vi "BASE_Parameters.vi"(8 "error in (no error)":errorcluster) -> (0 "error out":errorcluster)   [LabVIEW 2017]
doc: "this is Hardware setting to set ip address and com port of scanner"
uses:
  Global/PLC_to_Auto.vi
panel:
  in  "System Tab":T1(tab)
  in  "WRITE IN PLC":bool
  in  "MOTOR PARAMETERS":T2={"SPEED 1"=1000, "SPEED 2"=500, "SPEED 3"=100, "DISTANCE 1"=60.0, "DISTANCE 2"=5.0, "DISTANCE 3"=2.0, "MICRO STEP"=8, "STROKE COUNTER"=60} {"STROKE COUNTER" min=15 max=60 step=1; "MICRO STEP" min=1 max=3 step=1; "DISTANCE 3" min=0.5 max=2 step=0.1 format="%#.1g"; "DISTANCE 2" min=1 max=5 step=0.1 format="%#.1g"; "DISTANCE 1" min=40 max=60 step=0.1 format="%#.1g"; "SPEED 3" min=50 max=100 step=1; "SPEED 2" min=300 max=500 step=1; "SPEED 1" min=1000 max=2000 step=1}
  in  "TF CHECKING PARAMATERS":T3={"TRIP FORCE MIN"=40, "RESET FORCE MIN"=350, "OFFSET"=10, "TRIP FORCE MAX"=40, "RESET FORCE MAX"=350} {"RESET FORCE MAX" min=200 max=350 step=1; "TRIP FORCE MAX" min=15 max=40 step=1; "OFFSET" min=-10 max=10 step=1; "RESET FORCE MIN" min=200 max=350 step=1; "TRIP FORCE MIN" min=15 max=40 step=1}
  in  "Save Button":bool
  in  "Back":bool
  # "BARCODE VERIFICATION SYSTEM REPORTS"
  # "SPEED 1\t2000\nSPEED 2\t300\nSPEED 3\t100\nDISTANCE 1\t77.5 MM\nDISTANCE 2\t1.5 MM\nDISTANCE 3\t1.2 MM\nMEASURE BY MICRO\t5"
  # "Parameter Setting"
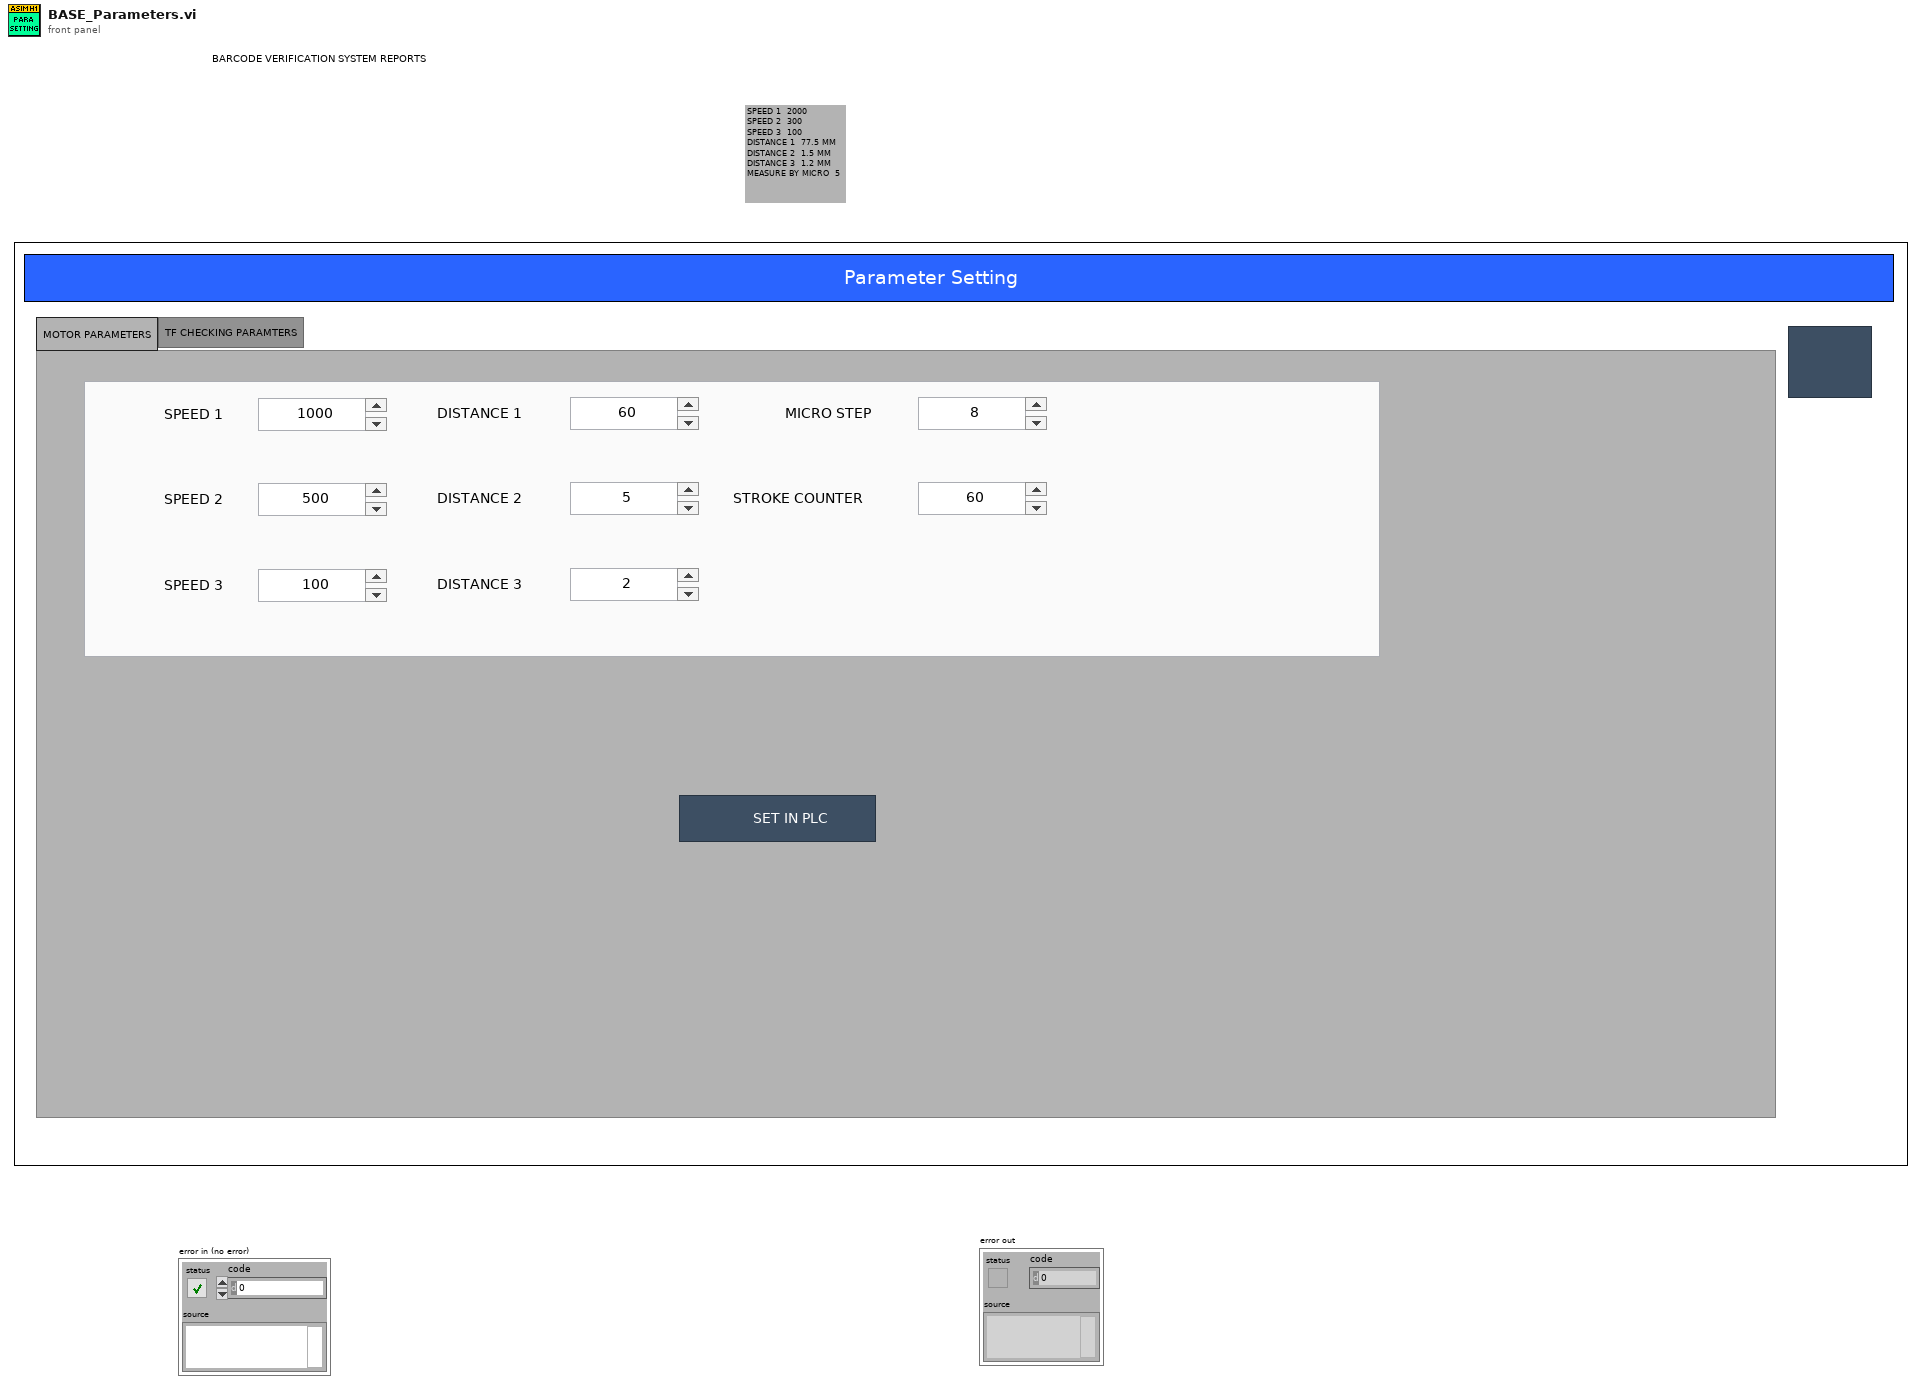
[diagram p1: front panel]
types:
  T1 = enum32{"MOTOR PARAMETERS", "TF CHECKING PARAMTERS"}
  T2 = cluster{"SPEED 1":u16, "SPEED 2":u16, "SPEED 3":u16, "DISTANCE 1":sgl, "DISTANCE 2":sgl, "DISTANCE 3":sgl, "MICRO STEP":u16, "STROKE COUNTER":u16}
  T3 = cluster{"TRIP FORCE MIN":u16, "RESET FORCE MIN":u16, "OFFSET":i16, "TRIP FORCE MAX":u16, "RESET FORCE MAX":u16}
  T4 = enum32{"invalid app kind", "Development System", "Run Time System", "Student Edition", "Embedded LabVIEW", "Evaluation", "Custom"}
  T5 = enum32{"Invalid", "Standard", "Closed", "Hidden", "Minimized", "Maximized"}
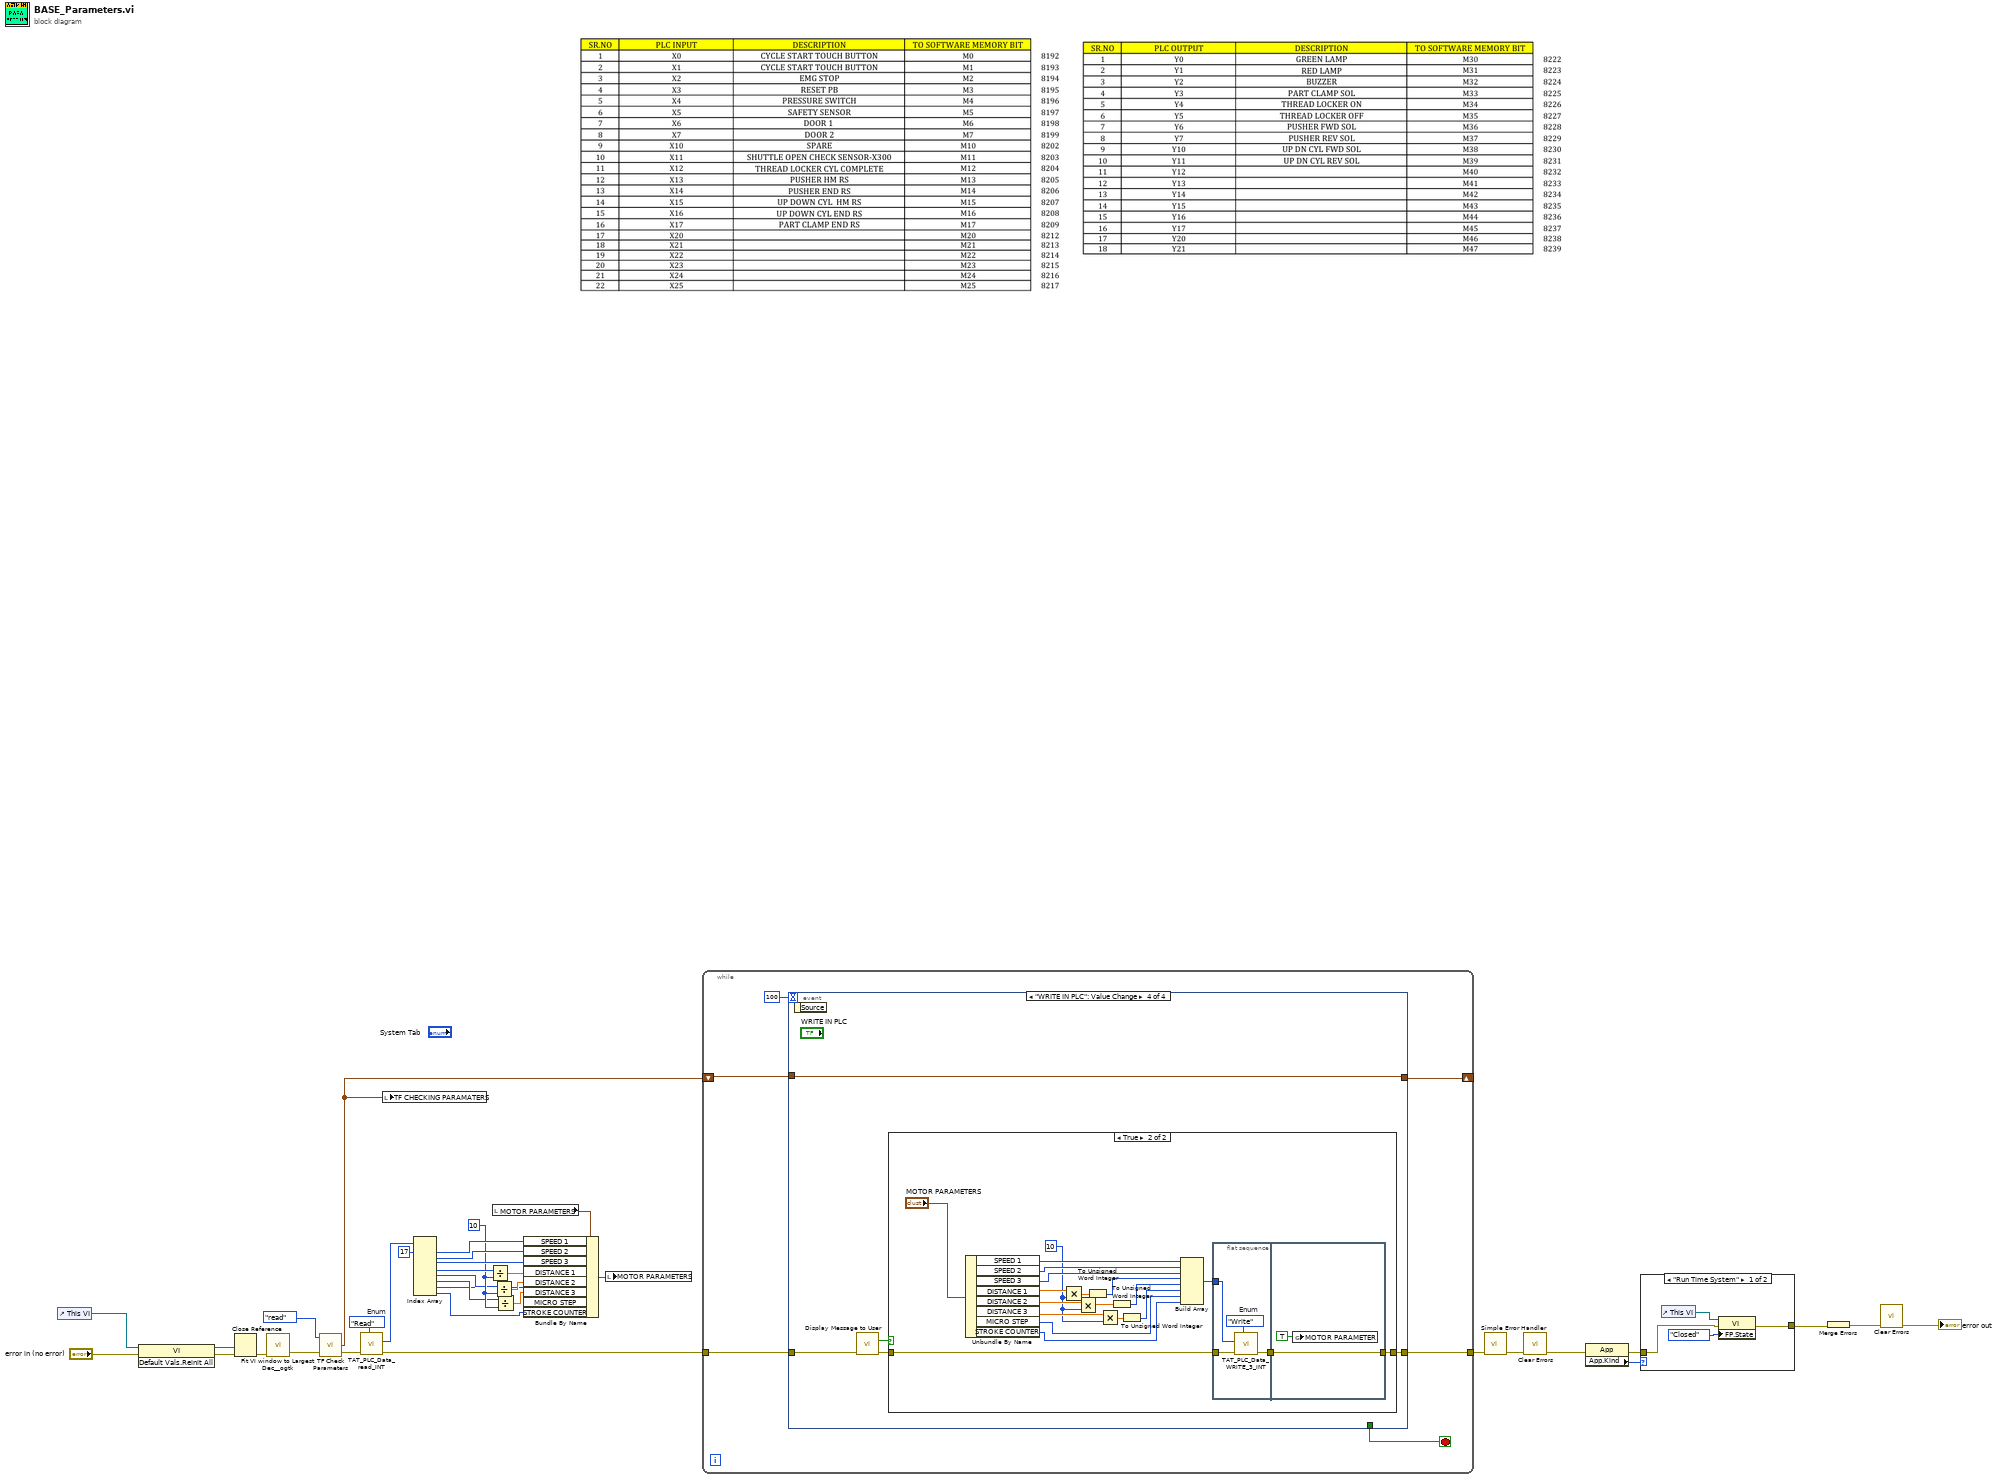
[diagram p0: block diagram]
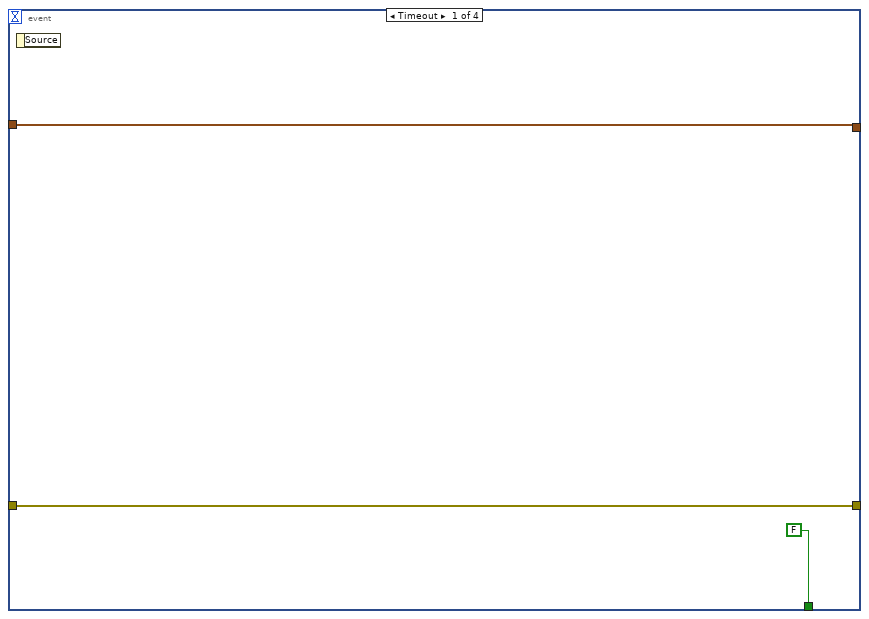
[diagram p2: hidden frame]
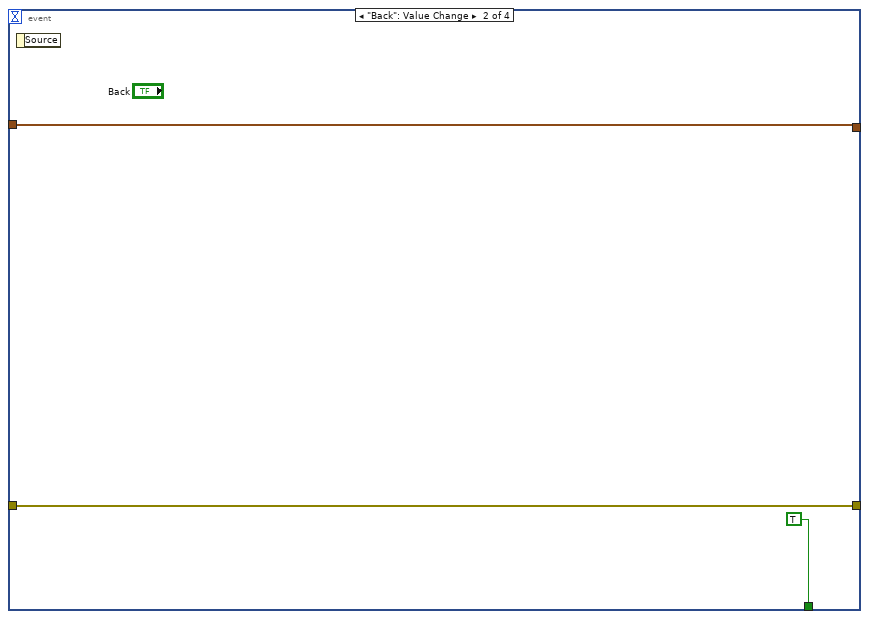
[diagram p3: hidden frame]
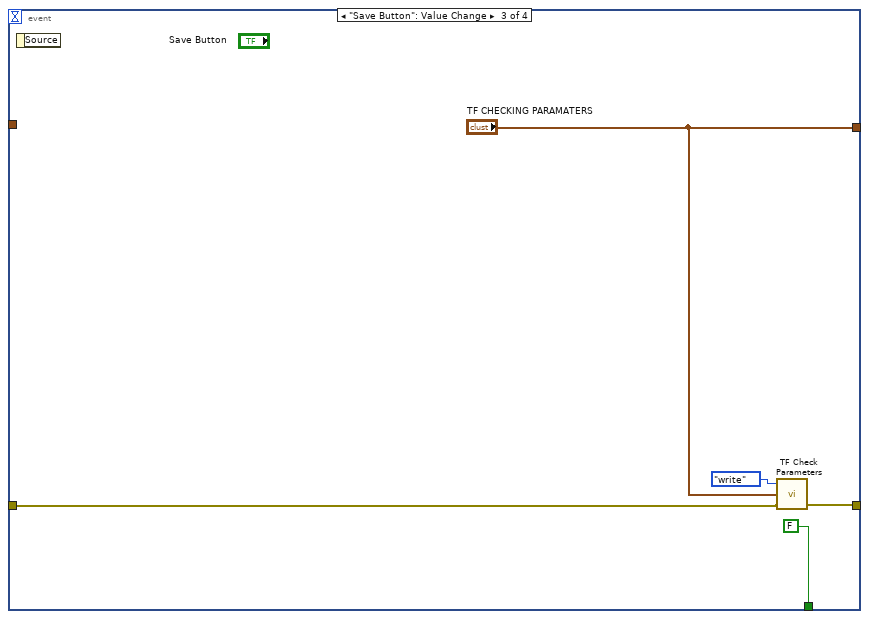
[diagram p4: hidden frame]
diagram:
  w7 = 10
  w19 = enum16{"Read", "Write"}."Read"  # Enum
  n1 = control-ref of="This VI"() -> (w32:refnum<vi>)
  n2 = invoke class="VI" method="Default Vals.Reinit All"(reference=w32, error in="error in (no error)") -> (reference out=w30:refnum<vi>, error out=w29:errorcluster)  [unwired: 1 in, 1 out]
  n3 = Close Reference(reference=w30, error in (no error)=w29) -> (error out=w28:errorcluster)
  n4 = call <userlib>:"Fit VI window to Largest Dec__ogtk.vi"("error in (no error)"=w28) -> ("error out"=w22:errorcluster)  [unwired: 5 in, 1 out]
  n5 = call "TF Check Parameters.vi"("error in"=w22, "Enum"=enum16{"read", "write"}."read") -> ("error our"=w18:errorcluster, "TF CHECKING PARAMATERS OUT"=w20:T3)  [unwired: 1 in, 1 out]
  n6 = call "TAT_PLC_Data_read_INT.vi"("Enum"=w19, "error in (no error)"=w18) -> ("error out"=w17:errorcluster, "Array 2"=w16:u16[])  [unwired: 8 in]
  n7 = local write "TF CHECKING PARAMATERS"(w20) -> ()
  n8 = Index Array(array=w16, index #1=17) -> (element #1=w14:u16, element #2=w13:u16, element #3=w12:u16, element #4=w11:u16, element #5=w6:u16, element #6=w5:u16, element #7=w4:u16, element #8=w3:u16)  [unwired: 7 in]
  n9 = Divide(x=w11, y=w7) -> (x/y=w10:dbl)
  n10 = local read "MOTOR PARAMETERS"() -> (w2:T2)
  n11 = Divide(x=w6, y=w7) -> (x/y=w9:dbl)
  n12 = Divide(x=w5, y=w7) -> (x/y=w8:dbl)
  n13 = Bundle By Name(cluster=w2, "SPEED 1"=w14, "SPEED 2"=w13, "SPEED 3"=w12, "DISTANCE 1"=w10, "DISTANCE 2"=w9, "DISTANCE 3"=w8, "MICRO STEP"=w4, "STROKE COUNTER"=w3) -> (w1:T2)
  n14 = local write "MOTOR PARAMETERS"(w1) -> ()
  n15 = while {
    tunnel: [w41] -> w23
    tunnel: w17 -> [w40]
    shift-right: [w39] -> _
    shift-left: w20 -> [w38]
    stop <- w36 stop-if-true
    n16 = event shown="[3] \"WRITE IN PLC\": Value Change" {
      selector: _ -> [_ _ _ _]
      dyn-events: _ -> [_ _ _ _]
      timeout: 100 -> [_ _ _ _]
      tunnel: [w42 w46 w50 w56] -> w41
      tunnel: w40 -> [w42 w46 w49 w55]
      tunnel: w38 -> [w44 w45 _ w57]
      tunnel: [w44 w45 "TF CHECKING PARAMATERS" w57] -> w39
      tunnel: [FALSE TRUE FALSE _] -> w36
      event Timeout {
        n17 = event-data() -> ()  [unwired: 1 in, 1 out]
      }
      event "Back": Value Change {
        n18 = event-data() -> ()  [unwired: 1 in, 1 out]
      }
      event "Save Button": Value Change {
        n19 = event-data() -> ()  [unwired: 1 in, 1 out]
        n20 = call "TF Check Parameters.vi"("error in"=w49, "TF CHECKING PARAMATERS IN"="TF CHECKING PARAMATERS", "Enum"=enum16{"read", "write"}."write") -> ("error our"=w50:errorcluster)  [unwired: 2 out]
      }
      event "WRITE IN PLC": Value Change {
        n21 = event-data() -> ()  [unwired: 1 in, 1 out]
        n22 = call "Display Message to User"("error in (no error)"=w55) -> ("error out"=w54:errorcluster, "OK"=w53:bool)  [unwired: 9 in]
        n23 = case shown="True" w53 {
          tunnel: w54 -> [w58 w60]
          tunnel: [w58 w59] -> w56
          frame False {
          }
          frame True {
            w71 = 10
            n24 = Unbundle By Name("MOTOR PARAMETERS") -> ("SPEED 1"=w77:u16, "SPEED 2"=w76:u16, "SPEED 3"=w75:u16, "DISTANCE 1"=w74:sgl, "DISTANCE 2"=w73:sgl, "DISTANCE 3"=w72:sgl, "MICRO STEP"=w64:u16, "STROKE COUNTER"=w63:u16)
            n25 = Multiply(x=w74, y=w71) -> (x*y=w70:sgl)
            n26 = Multiply(x=w73, y=w71) -> (x*y=w69:sgl)
            n27 = To Unsigned Word Integer(number=w70) -> (unsigned 16bit integer=w65:u16)
            n28 = Multiply(x=w72, y=w71) -> (x*y=w68:sgl)
            n29 = To Unsigned Word Integer(number=w69) -> (unsigned 16bit integer=w66:u16)
            n30 = To Unsigned Word Integer(number=w68) -> (unsigned 16bit integer=w67:u16)
            n31 = Build Array(w77, w76, w75, w65, w66, w67, w64, w63) -> (w61:u16[])
            n32 = flat-sequence {
              tunnel: w61 -> [w81]
              tunnel: w60 -> [w80]
              tunnel: [w79] -> w78
              tunnel: [w84] -> w59
              tunnel: w78 -> [w84]
              frame #0 {
                w82 = enum16{"Read", "Write"}."Write"  # Enum
                n33 = call "TAT_PLC_Data_WRITE_3_INT.vi"("Enum"=w82, "error in (no error)"=w80, "Array"=w81) -> ("error out"=w79:errorcluster)  [unwired: 7 in, 1 out]
              }
              frame #1 {
                n34 = global write "PLC_to_Auto.vi" "MOTOR PARAMETER"(TRUE) -> ()
              }
            }
          }
        }
      }
    }
  }
  n35 = call <vilib>:"Simple Error Handler.vi"("error in (no error)"=w23) -> ("error out"=w27:errorcluster)  [unwired: 4 in, 4 out]
  n36 = call <vilib>:"Clear Errors.vi"("error in (no error)"=w27) -> ("error out"=w24:errorcluster)  [unwired: 5 in, 1 out]
  n37 = property class="App"(error in=w24) -> (error out=w25:errorcluster, "App.Kind"=w26:T4)  [unwired: 1 in, 1 out]
  n38 = case shown="\"Run Time System\"" w26 {
    tunnel: w25 -> [w86 w89]
    tunnel: [w85 w89] -> w33
    frame "Run Time System" {
      n39 = control-ref of="This VI"() -> (w88:refnum<vi>)
      n40 = property class="VI"(reference=w88, error in=w86, "FP.State"=T5."Closed" ("Front Panel Window:State")) -> (error out=w85:errorcluster)  [unwired: 1 out]
    }
    frame "Development System", Default {
    }
  }
  n41 = Merge Errors(w33) -> (w34:errorcluster)
  n42 = call <vilib>:"Clear Errors.vi"("error in (no error)"=w34) -> ("error out"=→"error out":errorcluster)  [unwired: 5 in, 1 out]
